vi "DBtoArr.vi"() -> ()   [LabVIEW 2015]
uses:
  BERTTA.dll
panel:
  out "values":dbl[](array[numeric])
  in  "col":i32=4
  in  "nrows":i32=20
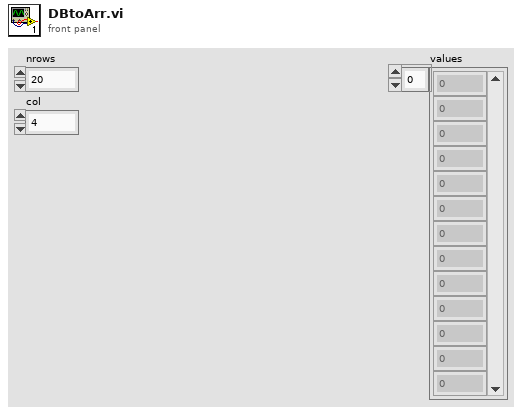
[diagram p1: front panel]
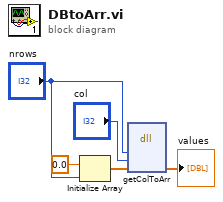
[diagram p0: block diagram]
diagram:
  n1 = Initialize Array(0.0 ("element"), "nrows") -> (w3:dbl[])
  n2 = dll-call lib="C:/Users/xlaraser/Documents/Visual Studio 2017/Projects/Bertta/BERTTA/Debug/BERTTA.dll" fn="getColToArr"("nrows"="nrows", "col"="col", "values"=w3) -> ("values"=→"values":dbl[])  [unwired: 6 in, 2 out]
